vi "Exemple_Metrics_Balanced_Accuracy_Score.vi"() -> ()   [LabVIEW 2020]
uses:
  Objet/3 - Model selection and evaluation/3.3 - Metrics and scoring/balanced_accuracy_score/Balanced_Accuracy_Score.vi
panel:
  out "Score":string
  out "error out":errorcluster caption="sortie d'erreur"
  in  "error in (no error)":errorcluster caption="entrée d'erreur (pas d'erreur)"
  in  "balanced_accuracy_score":cluster{"sample_weight":dbl[], "adjusted":bool}
  in  "y_pred":string[][](array[string])=[["0"], ["1"], ["0"], ["0"], ["0"], ["1"]]
  in  "y_true":string[][](array[string])=[["0"], ["1"], ["0"], ["0"], ["1"], ["0"]]
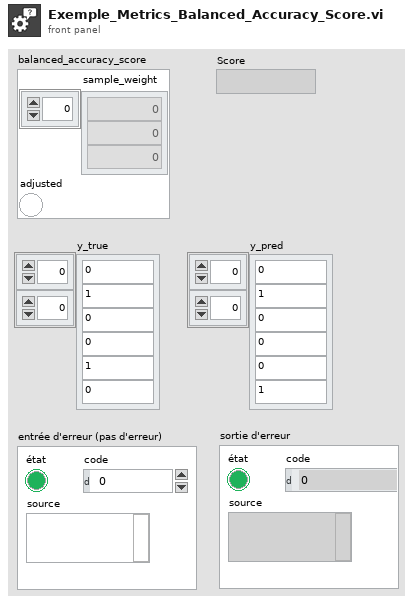
[diagram p1: front panel]
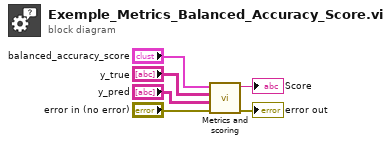
[diagram p0: block diagram]
diagram:
  n1 = call-poly "Metrics and scoring.vi"("error in (no error)"="error in (no error)", "y_pred"="y_pred", "y_true"="y_true", "balanced_accuracy_score"="balanced_accuracy_score") -> ("error out"=→"error out":errorcluster, "Score"=→"Score":string)  [unwired: 6 in]
